vi "GetCallers.vi"() -> (6 "Caller String":string)   [LabVIEW 2009]
doc: "Lists all callers of a VI in a \"f1->f2->....fn\" fashion."
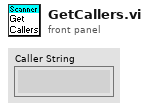
[diagram p1: front panel]
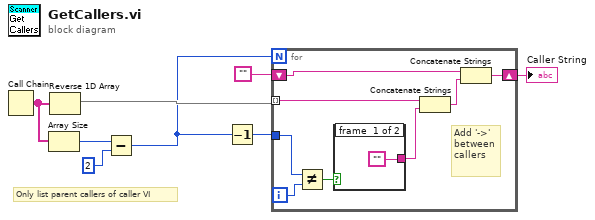
[diagram p0: block diagram]
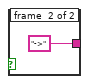
[diagram p2: hidden frame]
diagram:
  # "Only list parent callers of caller VI"
  n1 = Call Chain() -> (call chain=w7:string[])
  n2 = Array Size(array=w7) -> (size(s)=w2:i32)
  n3 = Reverse 1D Array(array=w7) -> (reversed array=w5:string[])
  n4 = Subtract(x=w2, y=2) -> (x-y=w4:i32)
  n5 = Decrement(x=w4) -> (x-1=w6:i32)
  n6 = for {
    N: w4 -> [_]
    tunnel: w5 -> [w16] mode=indexing
    shift-right: [w11] -> w3
    shift-left: "" -> [w10]
    tunnel: w6 -> [w9]
    i -> [w14]
    # "Add '->'\nbetween\ncallers"
    n7 = Not Equal?(x=w9, y=w14) -> (x != y?=w13:bool)
    n8 = case shown="True" w13 {
      tunnel: ["" "->" ("string")] -> w15
      frame #0 {
      }
      frame #1 {
      }
    }
    n9 = Concatenate Strings(w16, w15) -> (w12:string)
    n10 = Concatenate Strings(w10, w12) -> (w11:string)
  }
  "Caller String" <- w3
